vi "Remove Zeroes (2D String).vi"(8 "Array In":string[][](array[string])) -> (0 "Array Out":string[][](array[string]))   [LabVIEW 2013]
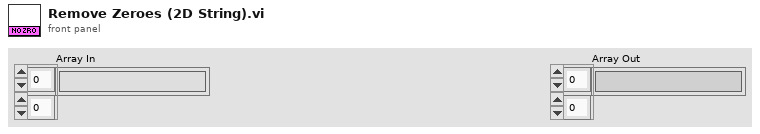
[diagram p1: front panel]
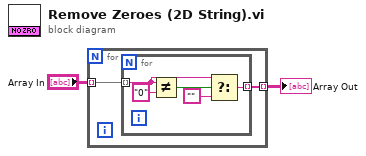
[diagram p0: block diagram]
diagram:
  n1 = for {
    tunnel: "Array In" -> [w4] mode=indexing
    tunnel: [w3] -> w1 mode=indexing
    n2 = for {
      tunnel: w4 -> [w7] mode=indexing
      tunnel: [w5] -> w3 mode=indexing
      n3 = Not Equal?(x=w7, y="0") -> (x != y?=w8:bool)
      n4 = Select(t=w7, s=w8, f="") -> (s? t:f=w5:string)
    }
  }
  "Array Out" <- w1
